vi "PHASE_OFFSET.vi"(0 "VISA IN":refnum<visa-resource-name>, 5 "error in":errorcluster) -> (14 "VISA Out":refnum<visa-resource-name>, 19 "error out":errorcluster)   [LabVIEW 2018, in "PNA-X.lvlib"]
uses:
  PNA-X.lvlib
panel:
  in  "Units for Phase":string(combo)="DEG"
  in  "Offset Phase Value":i32
  in  "Channel":i32=1
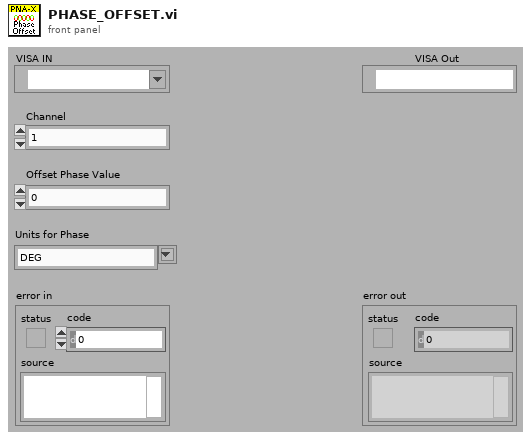
[diagram p1: front panel]
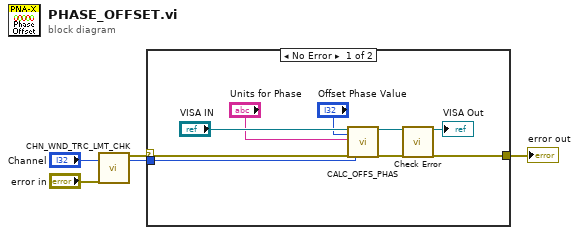
[diagram p0: block diagram]
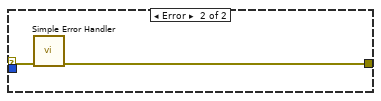
[diagram p2: hidden frame]
diagram:
  n1 = call "CHN_WND_TRC_LMT_CHK.vi"("Channel"="Channel", "error in"="error in") -> ("error out"=w2:errorcluster, "Channel"=w1:i32)  [unwired: 13 in, 3 out]
  n2 = case shown="No Error" w2 {
    selector: w2 -> [w12 w16]
    tunnel: [w14 w15] -> w4
    tunnel: w1 -> [w8 _]
    frame No Error {
      n3 = call "CALC_OFFS_PHAS.vi"("VISA IN"="VISA IN", "Offset Phase Value"="Offset Phase Value", "Units for Phase"="Units for Phase", "error in"=w12, "Channel"=w8) -> ("VISA Out"=w9:refnum<visa-resource-name>, "error out"=w11:errorcluster)  [unwired: 13 in]
      n4 = call "Check Error.vi"("VISA Resource Name"=w9, "error in (no error)"=w11) -> ("dup VISA session"=→"VISA Out":refnum<visa-resource-name>, "error out"=w14:errorcluster)  [unwired: 16 in]
    }
    frame Error {
      n5 = call <vilib>:"Simple Error Handler.vi"("error in (no error)"=w16) -> ("error out"=w15:errorcluster)  [unwired: 4 in, 4 out]
    }
  }
  "error out" <- w4
